vi "Next move.vi"(9 "Elevator states in":T1[](array[typedef])=[{"Elevator"={"Up Button"=FALSE, "Current floor"=1, "Down Button"=FALSE, "Car"={"Blank Button"=FALSE, "Blank Button 2"=FALSE, "Blank Button 3"=FALSE, "Blank Button 4"=FALSE, "Blank Button 5"=FALSE, "Blank Button 6"=FALSE, "Blank Button 7"=FALSE, "Blank Button 8"=FALSE, "Blank Button 9"=FALSE, "Blank Button 10"=FALSE, "Blank Button 11"=FALSE, "Blank Button 12"=FALSE, "Blank Button 13"=FALSE, "Blank Button 14"=FALSE, "Blank Button 15"=FALSE, "Blank Button 16"=FALSE, "Blank Button 17"=FALSE, "Blank Button 18"=FALSE, "Blank Button 19"=FALSE, "Blank Button 20"=FALSE}, "Close door"=FALSE}, "Destinations"=[], "Idle floor"=1, "Max floor"=7, "Min floor"=1, "Next floor"=0, "Move started"=timestamp(0 s since 1904-01-01), "Idle move"=FALSE}, {"Elevator"={"Up Button"=FALSE, "Current floor"=8, "Down Button"=FALSE, "Car"={"Blank Button"=FALSE, "Blank Button 2"=FALSE, "Blank Button 3"=FALSE, "Blank Button 4"=FALSE, "Blank Button 5"=FALSE, "Blank Button 6"=FALSE, "Blank Button 7"=FALSE, "Blank Button 8"=FALSE, "Blank Button 9"=FALSE, "Blank Button 10"=FALSE, "Blank Button 11"=FALSE, "Blank Button 12"=FALSE, "Blank Button 13"=FALSE, "Blank Button 14"=FALSE, "Blank Button 15"=FALSE, "Blank Button 16"=FALSE, "Blank Button 17"=FALSE, "Blank Button 18"=FALSE, "Blank Button 19"=FALSE, "Blank Button 20"=FALSE}, "Close door"=FALSE}, "Destinations"=[], "Idle floor"=8, "Max floor"=14, "Min floor"=8, "Next floor"=0, "Move started"=timestamp(0 s since 1904-01-01), "Idle move"=FALSE}, {"Elevator"={"Up Button"=FALSE, "Current floor"=1, "Down Button"=FALSE, "Car"={"Blank Button"=FALSE, "Blank Button 2"=FALSE, "Blank Button 3"=FALSE, "Blank Button 4"=FALSE, "Blank Button 5"=FALSE, "Blank Button 6"=FALSE, "Blank Button 7"=FALSE, "Blank Button 8"=FALSE, "Blank Button 9"=FALSE, "Blank Button 10"=FALSE, "Blank Button 11"=FALSE, "Blank Button 12"=FALSE, "Blank Button 13"=FALSE, "Blank Button 14"=FALSE, "Blank Button 15"=FALSE, "Blank Button 16"=FALSE, "Blank Button 17"=FALSE, "Blank Button 18"=FALSE, "Blank Button 19"=FALSE, "Blank Button 20"=FALSE}, "Close door"=FALSE}, "Destinations"=[], "Idle floor"=1, "Max floor"=14, "Min floor"=1, "Next floor"=0, "Move started"=timestamp(0 s since 1904-01-01), "Idle move"=FALSE}, {"Elevator"={"Up Button"=FALSE, "Current floor"=14, "Down Button"=FALSE, "Car"={"Blank Button"=FALSE, "Blank Button 2"=FALSE, "Blank Button 3"=FALSE, "Blank Button 4"=FALSE, "Blank Button 5"=FALSE, "Blank Button 6"=FALSE, "Blank Button 7"=FALSE, "Blank Button 8"=FALSE, "Blank Button 9"=FALSE, "Blank Button 10"=FALSE, "Blank Button 11"=FALSE, "Blank Button 12"=FALSE, "Blank Button 13"=FALSE, "Blank Button 14"=FALSE, "Blank Button 15"=FALSE, "Blank Button 16"=FALSE, "Blank Button 17"=FALSE, "Blank Button 18"=FALSE, "Blank Button 19"=FALSE, "Blank Button 20"=FALSE}, "Close door"=FALSE}, "Destinations"=[], "Idle floor"=14, "Max floor"=20, "Min floor"=6, "Next floor"=0, "Move started"=timestamp(0 s since 1904-01-01), "Idle move"=FALSE}]) -> (1 "Elevator states out":T1[](array[typedef])=[{"Elevator"={"Up Button"=FALSE, "Current floor"=1, "Down Button"=FALSE, "Car"={"Blank Button"=FALSE, "Blank Button 2"=FALSE, "Blank Button 3"=FALSE, "Blank Button 4"=FALSE, "Blank Button 5"=FALSE, "Blank Button 6"=FALSE, "Blank Button 7"=FALSE, "Blank Button 8"=FALSE, "Blank Button 9"=FALSE, "Blank Button 10"=FALSE, "Blank Button 11"=FALSE, "Blank Button 12"=FALSE, "Blank Button 13"=FALSE, "Blank Button 14"=FALSE, "Blank Button 15"=FALSE, "Blank Button 16"=FALSE, "Blank Button 17"=FALSE, "Blank Button 18"=FALSE, "Blank Button 19"=FALSE, "Blank Button 20"=FALSE}, "Close door"=FALSE}, "Destinations"=[], "Idle floor"=1, "Max floor"=7, "Min floor"=1, "Next floor"=0, "Move started"=timestamp(0 s since 1904-01-01), "Idle move"=FALSE}, {"Elevator"={"Up Button"=FALSE, "Current floor"=8, "Down Button"=FALSE, "Car"={"Blank Button"=FALSE, "Blank Button 2"=FALSE, "Blank Button 3"=FALSE, "Blank Button 4"=FALSE, "Blank Button 5"=FALSE, "Blank Button 6"=FALSE, "Blank Button 7"=FALSE, "Blank Button 8"=FALSE, "Blank Button 9"=FALSE, "Blank Button 10"=FALSE, "Blank Button 11"=FALSE, "Blank Button 12"=FALSE, "Blank Button 13"=FALSE, "Blank Button 14"=FALSE, "Blank Button 15"=FALSE, "Blank Button 16"=FALSE, "Blank Button 17"=FALSE, "Blank Button 18"=FALSE, "Blank Button 19"=FALSE, "Blank Button 20"=FALSE}, "Close door"=FALSE}, "Destinations"=[], "Idle floor"=8, "Max floor"=14, "Min floor"=8, "Next floor"=0, "Move started"=timestamp(0 s since 1904-01-01), "Idle move"=FALSE}, {"Elevator"={"Up Button"=FALSE, "Current floor"=1, "Down Button"=FALSE, "Car"={"Blank Button"=FALSE, "Blank Button 2"=FALSE, "Blank Button 3"=FALSE, "Blank Button 4"=FALSE, "Blank Button 5"=FALSE, "Blank Button 6"=FALSE, "Blank Button 7"=FALSE, "Blank Button 8"=FALSE, "Blank Button 9"=FALSE, "Blank Button 10"=FALSE, "Blank Button 11"=FALSE, "Blank Button 12"=FALSE, "Blank Button 13"=FALSE, "Blank Button 14"=FALSE, "Blank Button 15"=FALSE, "Blank Button 16"=FALSE, "Blank Button 17"=FALSE, "Blank Button 18"=FALSE, "Blank Button 19"=FALSE, "Blank Button 20"=FALSE}, "Close door"=FALSE}, "Destinations"=[], "Idle floor"=1, "Max floor"=14, "Min floor"=1, "Next floor"=0, "Move started"=timestamp(0 s since 1904-01-01), "Idle move"=FALSE}, {"Elevator"={"Up Button"=FALSE, "Current floor"=14, "Down Button"=FALSE, "Car"={"Blank Button"=FALSE, "Blank Button 2"=FALSE, "Blank Button 3"=FALSE, "Blank Button 4"=FALSE, "Blank Button 5"=FALSE, "Blank Button 6"=FALSE, "Blank Button 7"=FALSE, "Blank Button 8"=FALSE, "Blank Button 9"=FALSE, "Blank Button 10"=FALSE, "Blank Button 11"=FALSE, "Blank Button 12"=FALSE, "Blank Button 13"=FALSE, "Blank Button 14"=FALSE, "Blank Button 15"=FALSE, "Blank Button 16"=FALSE, "Blank Button 17"=FALSE, "Blank Button 18"=FALSE, "Blank Button 19"=FALSE, "Blank Button 20"=FALSE}, "Close door"=FALSE}, "Destinations"=[], "Idle floor"=14, "Max floor"=20, "Min floor"=6, "Next floor"=0, "Move started"=timestamp(0 s since 1904-01-01), "Idle move"=FALSE}], 2 "Served floors":u16[](array[numeric]), 5 "Served car":bool[](array[boolean]))   [LabVIEW 2019]
uses:
  Type defs/Elevator states.ctl
  Type defs/Elevator position.ctl
  Type defs/Car buttons.ctl
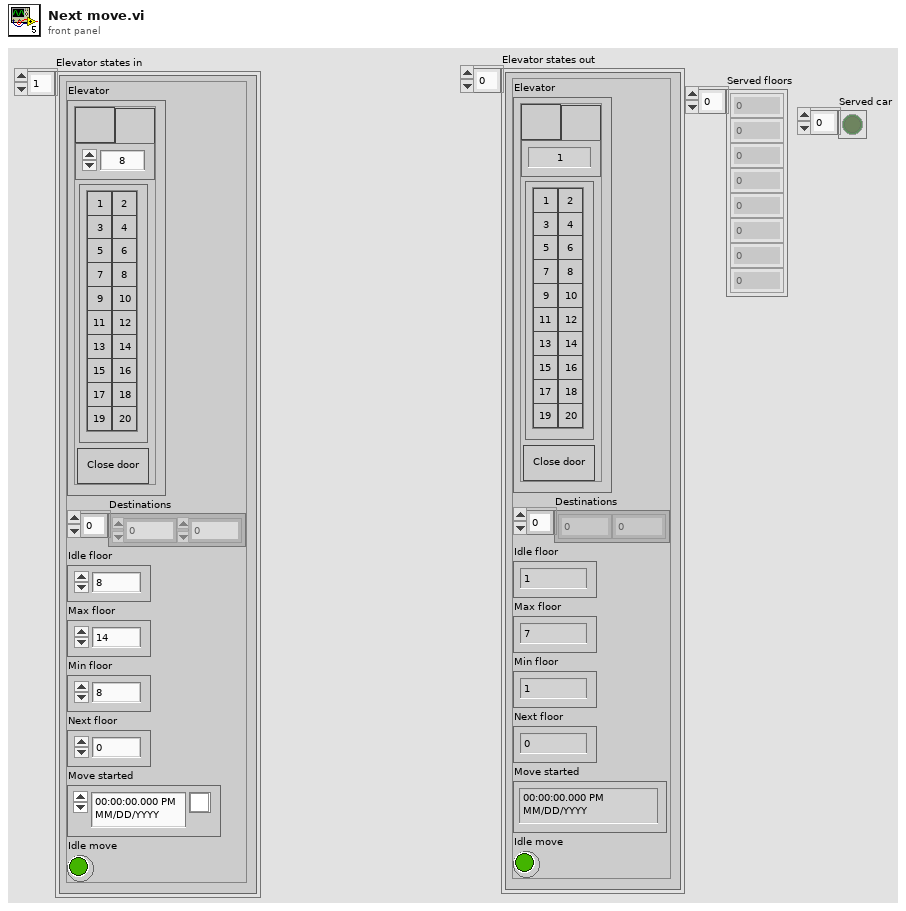
[diagram p1: front panel]
types:
  T1 = typedef "Elevator states.ctl" = cluster{"Elevator":T2, "Destinations":i32[], "Idle floor":u16, "Max floor":u16, "Min floor":u16, "Next floor":u16, "Move started":timestamp, "Idle move":bool}
  T2 = typedef "Elevator position.ctl" = cluster{"Up Button":bool, "Current floor":u16, "Down Button":bool, "Car":T3, "Close door":bool}
  T3 = typedef "Car buttons.ctl" = cluster{"Blank Button":bool, "Blank Button 2":bool, "Blank Button 3":bool, "Blank Button 4":bool, "Blank Button 5":bool, "Blank Button 6":bool, "Blank Button 7":bool, "Blank Button 8":bool, "Blank Button 9":bool, "Blank Button 10":bool, "Blank Button 11":bool, "Blank Button 12":bool, "Blank Button 13":bool, "Blank Button 14":bool, "Blank Button 15":bool, "Blank Button 16":bool, "Blank Button 17":bool, "Blank Button 18":bool, "Blank Button 19":bool, "Blank Button 20":bool}
  T4 = cluster{"Car[0]":bool, "Car[1]":bool, "Car[2]":bool, "Car[3]":bool, "Car[4]":bool, "Car[5]":bool, "Car[6]":bool, "Car[7]":bool, "Car[8]":bool, "Car[9]":bool, "Car[10]":bool, "Car[11]":bool, "Car[12]":bool, "Car[13]":bool, "Car[14]":bool, "Car[15]":bool, "Car[16]":bool, "Car[17]":bool, "Car[18]":bool, "Car[19]":bool}
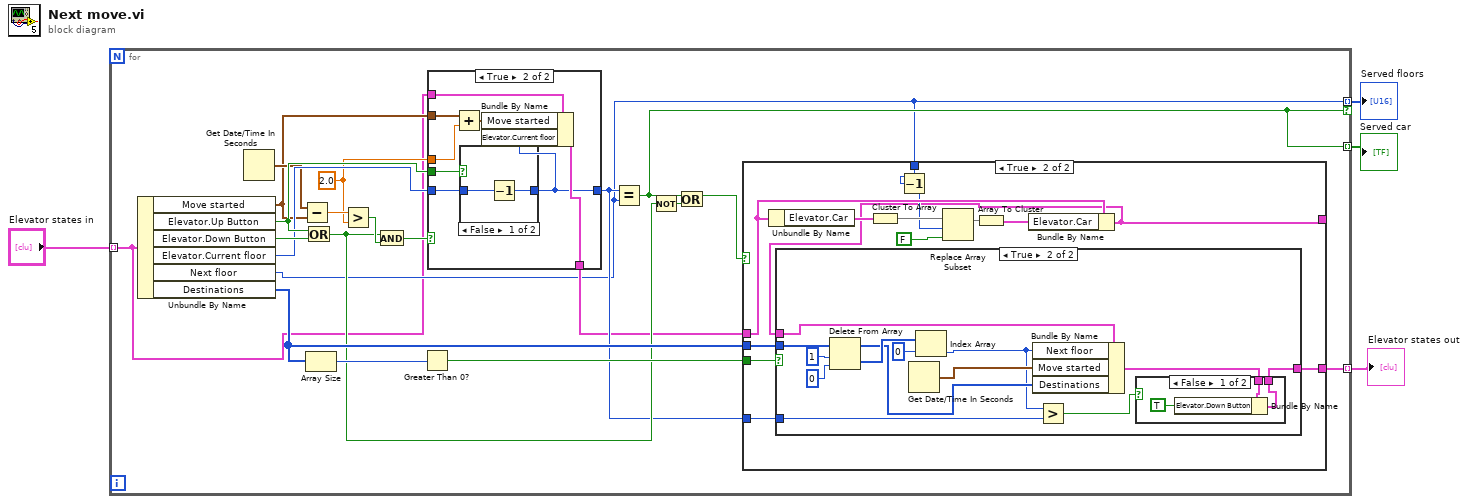
[diagram p0: block diagram]
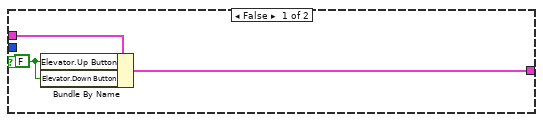
[diagram p3: hidden frame]
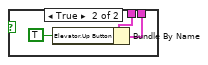
[diagram p4: hidden frame]
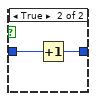
[diagram p6: hidden frame]
diagram:
  n1 = for {
    tunnel: "Elevator states in" -> [w5] mode=indexing
    tunnel: [w13] -> w3 mode=indexing
    tunnel: [w6] -> w2 mode=indexing if=w7
    tunnel: [w7] -> w1 mode=indexing
    w17 = 2.0 ("y")
    n2 = Unbundle By Name(w5) -> ("Move started"=w18:timestamp, "Elevator.Up Button"=w23:bool, "Elevator.Down Button"=w25:bool, "Elevator.Current floor"=w22:u16, "Next floor"=w6:u16, "Destinations"=w14:i32[])
    n3 = Get Date/Time In Seconds() -> (seconds since 1Jan1904=w21:timestamp)
    n4 = Subtract(x=w21, y=w18) -> (x-y=w20:dbl)
    n5 = Or(x=w23, y=w25) -> (x .or. y?=w11:bool)
    n6 = Array Size(array=w14) -> (size(s)=w16:i32)
    n7 = Greater?(x=w20, y=w17) -> (0:w19:bool)
    n8 = And(x=w11, y=w19) -> (x .and. y?=w24:bool)
    n9 = Greater Than 0?(x=w16) -> (x > 0?=w15:bool)
    n10 = case shown="True" w24 {
      tunnel: w23 -> [_ w71]
      tunnel: w22 -> [w63 w70]
      tunnel: [w63 w64] -> w9
      tunnel: w5 -> [w62 w69]
      tunnel: w18 -> [_ w68]
      tunnel: w17 -> [_ w67]
      tunnel: [w62 w65] -> w8
      frame False {
      }
      frame True {
        n11 = Add(x=w68, y=w67) -> (x+y=w66:timestamp)
        n12 = case shown="False" w71 {
          tunnel: w70 -> [w73 w75]
          tunnel: [w72 w74] -> w64
          frame False {
            n13 = Decrement(x=w73) -> (x-1=w72:u16)
          }
          frame True {
            n14 = Increment(x=w75) -> (x+1=w74:u16)
          }
        }
        n15 = Bundle By Name(cluster=w69, "Move started"=w66, "Elevator.Current floor"=w64) -> (w65:T1)
      }
    }
    n16 = Equal?(x=w9, y=w6) -> (x = y?=w7:bool)
    n17 = Not(x=w11) -> (.not. x?=w10:bool)
    n18 = Or(x=w7, y=w10) -> (x .or. y?=w12:bool)
    n19 = case shown="True" w12 {
      tunnel: w15 -> [_ w39]
      tunnel: w14 -> [_ w38]
      tunnel: w8 -> [w26 w30]
      tunnel: [w26 w37] -> w13
      tunnel: w9 -> [_ w36]
      tunnel: w6 -> [_ w32]
      tunnel: [_ w27] -> _
      frame False {
      }
      frame True {
        n20 = Unbundle By Name(w30) -> ("Elevator.Car"=w35:T3)
        n21 = Cluster To Array(cluster=w35) -> (array=w34:bool[])
        n22 = Decrement(x=w32) -> (x-1=w28:u16)
        n23 = Replace Array Subset(array=w34, new element=FALSE ("new element/subarray"), index=w28) -> (w31:bool[])
        n24 = Array To Cluster(array=w31) -> (cluster=w29:T4)
        n25 = Bundle By Name(cluster=w30, "Elevator.Car"=w29) -> (w27:T1)
        n26 = case shown="True" w39 {
          tunnel: w38 -> [_ w55]
          tunnel: w27 -> [w42 w50]
          tunnel: [w40 w43] -> w37
          tunnel: w36 -> [_ w46]
          frame False {
            w41 = FALSE ("Elevator.Up Button")
            n27 = Bundle By Name(cluster=w42, "Elevator.Up Button"=w41, "Elevator.Down Button"=w41) -> (w40:T1)
          }
          frame True {
            n28 = Delete From Array(array=w55, length=1, index=0) -> (deleted portion=w52:i32[], array with subset deleted=w48:i32[])
            n29 = Get Date/Time In Seconds() -> (seconds since 1Jan1904=w49:timestamp)
            n30 = Index Array(array=w52, index=0) -> (element=w47:i32)
            n31 = Bundle By Name(cluster=w50, "Next floor"=w47, "Move started"=w49, "Destinations"=w48) -> (w44:T1)
            n32 = Greater?(x=w47, y=w46) -> (0:w45:bool)
            n33 = case shown="False" w45 {
              tunnel: w44 -> [w58 w61]
              tunnel: [w57 w59] -> w43
              frame False {
                n34 = Bundle By Name(cluster=w58, "Elevator.Down Button"=TRUE) -> (w57:T1)
              }
              frame True {
                n35 = Bundle By Name(cluster=w61, "Elevator.Up Button"=TRUE) -> (w59:T1)
              }
            }
          }
        }
      }
    }
  }
  "Elevator states out" <- w3
  "Served floors" <- w2
  "Served car" <- w1
